vi "Move-For-Distance-Subtask1.vi"() -> ()   [LabVIEW 2016, in "LEGO-PMR.lvrbt"]
uses:
  LEGO-PMR.lvrbt
  <vilib>/NXT/Block Support/NXT_OutputPort.ctl
  <vilib>/NXT/LegoClasses/BrickReference/BrickReference.lvclass
  <vilib>/NXT/Subs/LVHSConnector.ctl
  <vilib>/NXT/NXTIO Xnodes/NXTIOXNode/NXTIO.xnode
  <vilib>/NXT/NXTIO Xnodes/AddressXNode/NXTIOAddress.xnode
  <vilib>/NXT/Dual Mode Library/Waits/Wait_Num.vi
  <vilib>/NXT/NXTIO Xnodes/NXTIONodeSubVIs/NXTMoveMotors.vi
panel:
  in  "Distance (in Inches)":dbl
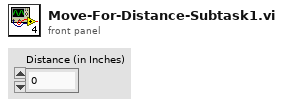
[diagram p1: front panel]
types:
  T1 = typedef "LVHSConnector.ctl" = refnum<class "BrickReference.lvclass">
  T2 = typedef "NXT_OutputPort.ctl" = u8
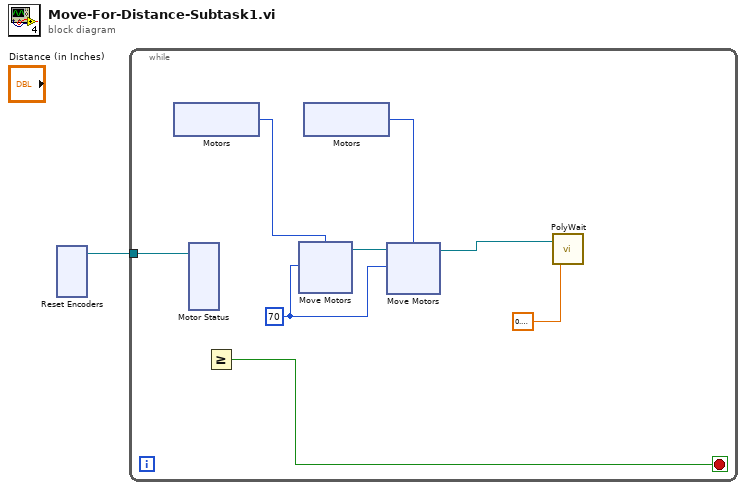
[diagram p0: block diagram]
diagram:
  n1 = xnode "Reset Encoders"() -> ("NXT/EV3"=w1:T1)  [unwired: 2 in]
  n2 = while {
    tunnel: w1 -> [w5]
    stop <- w8 stop-if-true
    w2 = 70
    n3 = xnode "Motors"() -> ("Motor"=w7:T2)
    n4 = xnode "Motor Status"("NXT/EV3"=w5) -> ()  [unwired: 1 in, 3 out]
    n5 = Greater Or Equal?() -> (x >= y?=w8:bool)  [unwired: 2 in]
    n6 = xnode "Move Motors"("Power/Speed 1"=w2, "Motors"=w7) -> ("NXT/EV3"=w4:T1)  [unwired: 1 in]
    n7 = xnode "Motors"() -> ("Motor"=w6:T2)
    n8 = xnode "Move Motors"("Power/Speed 1"=w2, "Motors"=w6, "NXT/EV3"=w4) -> ("NXT/EV3"=w3:T1)
    n9 = call-poly <vilib>:"PolyWait.vi"("Time (1 sec)"=0.10000000000000002, "NXT/EV3"=w3) -> ()  [unwired: 2 in, 1 out]
  }
